vi "diff_x1.vi"() -> ()   [LabVIEW 2014]
panel:
  in  "diff_x1":dbl
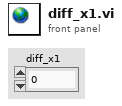
[diagram p1: front panel]
diagram:
